vi "Facade.vi"(0 "Data In":T4, 2 "Display State In":T2, 3 "Container State":T3) -> (6 "Data Out":T4, 7 "Display State Out":T2, 8 "Action":T1)   [LabVIEW 2015, in "Moving Ripple Noise.xctl"]
uses:
  Moving Ripple Noise.xctl
  Data.vi
  Classes/Waveforms/Moving Ripple Noise/Moving Ripple Noise.lvclass
  <vilib>/_xctls/Container State.ctl
  State.vi
  <vilib>/_xctls/Action.ctl
  Classes/Waveforms/Moving Ripple Noise/Moving Ripple Noise.lvclass/Moving Ripple Noise.ctl
  Classes/Waveforms/Moving Ripple Noise/Read Fmin.vi
  Classes/Waveforms/Moving Ripple Noise/Read Fmax.vi
  Classes/Waveforms/Moving Ripple Noise/Read Comp_oct.vi
  Classes/Waveforms/Moving Ripple Noise/Read Density.vi
  Classes/Waveforms/Moving Ripple Noise/Read Velocity.vi
  Classes/Waveforms/Moving Ripple Noise/Read Depth.vi
  Classes/Waveforms/Moving Ripple Noise/Read Phase.vi
  Classes/Waveforms/Moving Ripple Noise/Write Fmin.vi
  Classes/Waveforms/Moving Ripple Noise/Write Fmax.vi
  Classes/Waveforms/Moving Ripple Noise/Write Comp_oct.vi
  Classes/Waveforms/Moving Ripple Noise/Write Density.vi
  Classes/Waveforms/Moving Ripple Noise/Write Velocity.vi
  Classes/Waveforms/Moving Ripple Noise/Write Depth.vi
  Classes/Waveforms/Moving Ripple Noise/Write Phase.vi
  <vilib>/_xctls/XControlSupport.lvlib
panel:
  in  "Plot":bool
  in  "Comp/oct":i32
  in  "Depth (0-1)":dbl
  in  "Velocity (Hz)":dbl
  in  "Density (cyc/oct)":dbl
  in  "Phase (cyc)":dbl
  in  "Fmin (Hz)":dbl
  in  "Fmax (Hz)":dbl
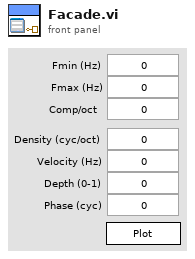
[diagram p1: front panel]
types:
  T1 = typedef "XControlSupport.lvlib/Action.ctl" = cluster{"Data Changed?":bool, "State Changed?":bool, "Action Name":string}
  T2 = typedef "Moving Ripple Noise.xctl/State.vi" = cluster{"Numeric":dbl}
  T3 = typedef "XControlSupport.lvlib/Container State.ctl" = cluster{"Indicator?":bool, "Run Mode?":bool, " Refnum":refnum<vi>}
  T4 = typedef "Moving Ripple Noise.xctl/Data.vi" = refnum<class "Moving Ripple Noise.lvclass">
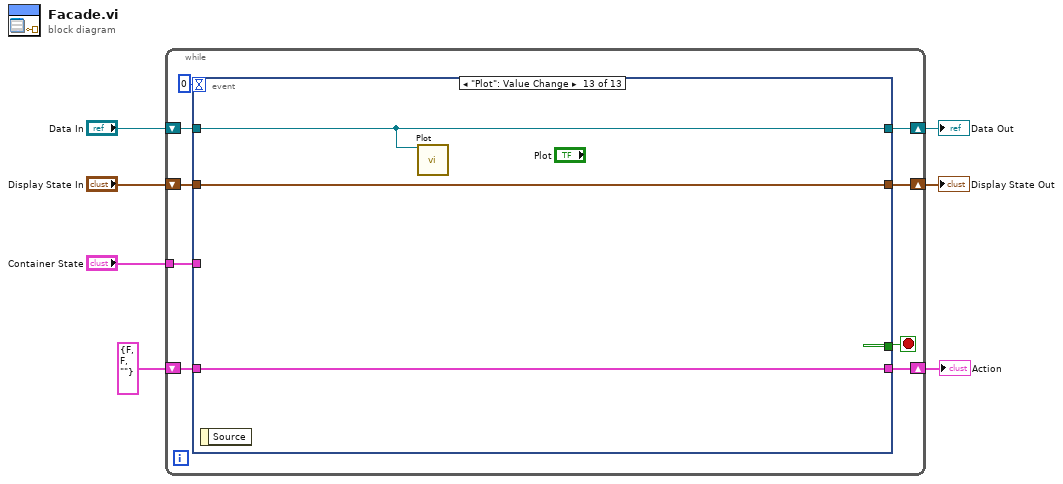
[diagram p0: block diagram]
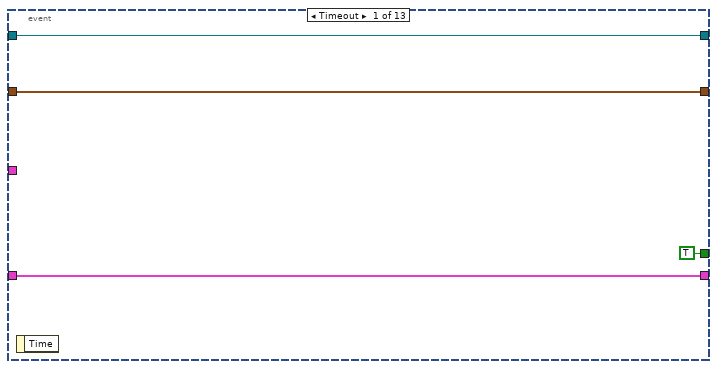
[diagram p2: hidden frame]
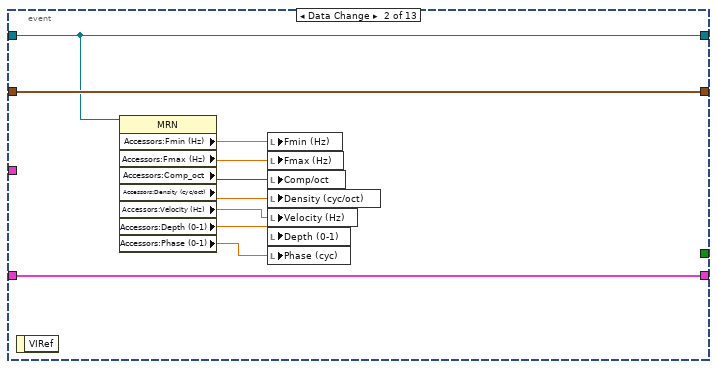
[diagram p3: hidden frame]
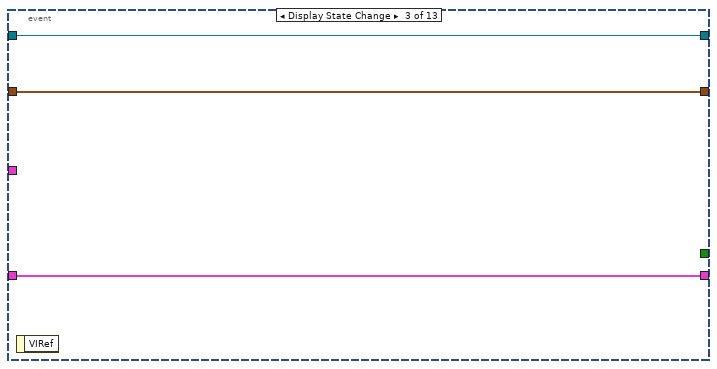
[diagram p4: hidden frame]
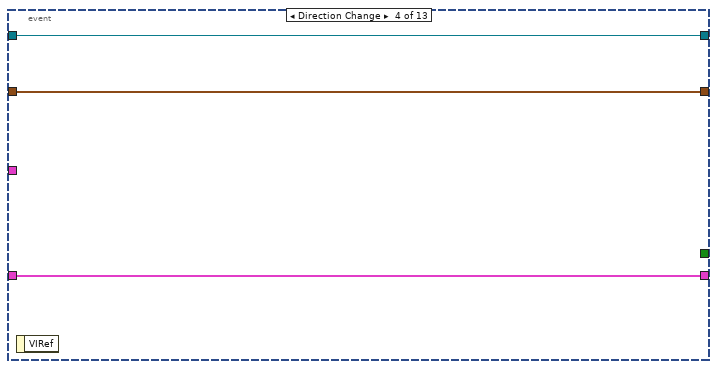
[diagram p5: hidden frame]
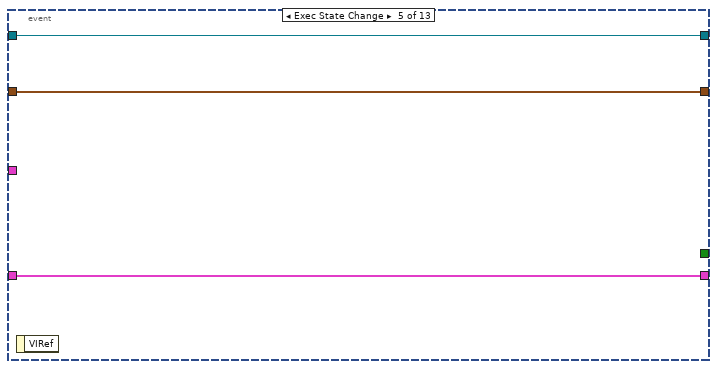
[diagram p6: hidden frame]
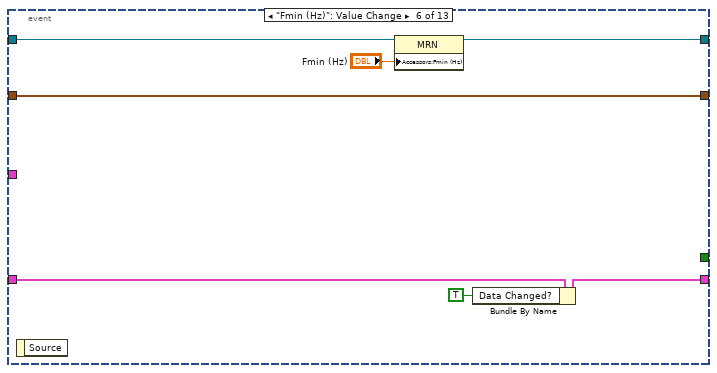
[diagram p7: hidden frame]
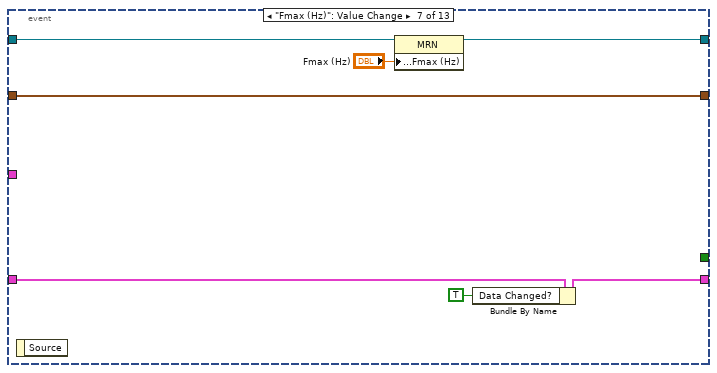
[diagram p8: hidden frame]
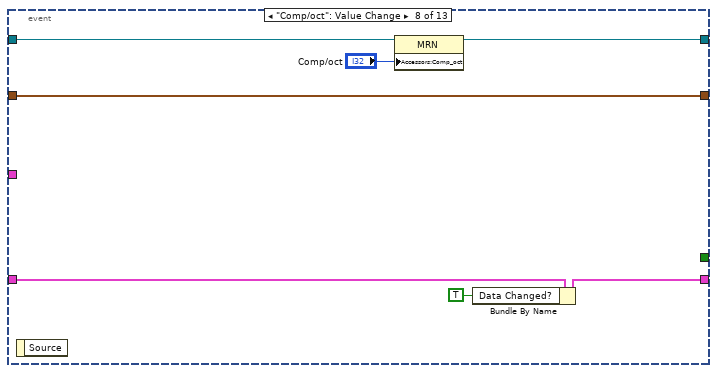
[diagram p9: hidden frame]
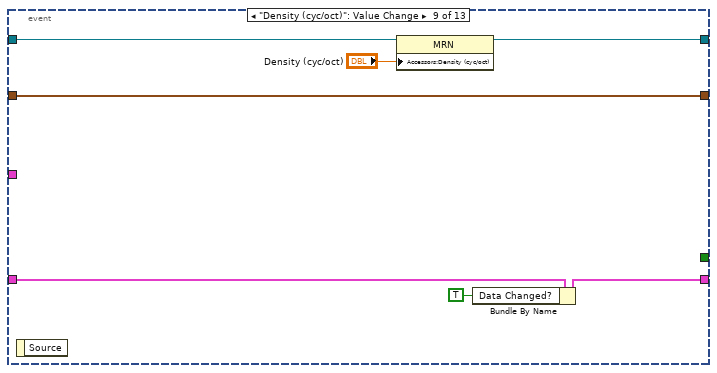
[diagram p10: hidden frame]
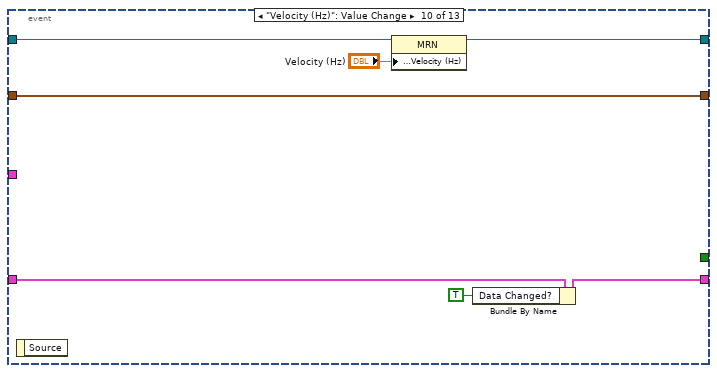
[diagram p11: hidden frame]
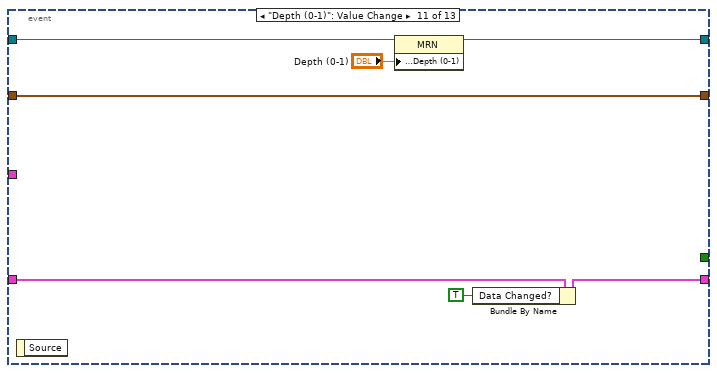
[diagram p12: hidden frame]
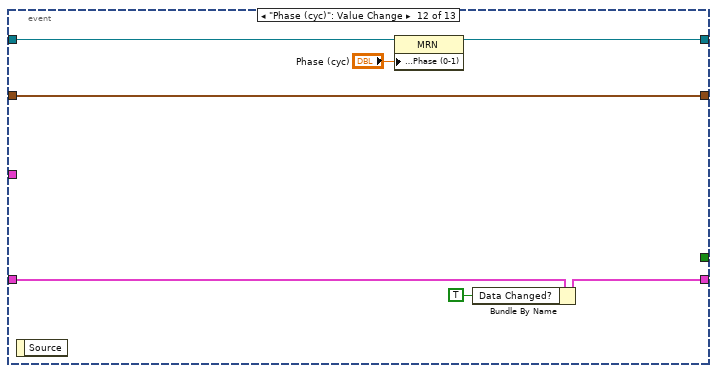
[diagram p13: hidden frame]
diagram:
  n1 = while {
    shift-right: [w15] -> w4
    shift-left: "Display State In" -> [w16]
    tunnel: "Container State" -> [w12]
    shift-right: [w10] -> w7
    shift-left: "Data In" -> [w11]
    shift-right: [w8] -> w2
    shift-left: T1 {"Data Changed?"=FALSE, "State Changed?"=FALSE, "Action Name"=""} ("Action") -> [w9]
    stop <- w14 stop-if-true
    n2 = event shown="[12] \"Plot\": Value Change" {
      selector: _ -> [_ _ _ _ _ _ _ _ _ _ _ _ _]
      dyn-events: _ -> [_ _ _ _ _ _ _ _ _ _ _ _ _]
      timeout: 0 -> [_ _ _ _ _ _ _ _ _ _ _ _ _]
      tunnel: w16 -> [w18 w30 w33 w36 w39 w46 w53 w60 w67 w74 w81 w88 w91]
      tunnel: [w18 w30 w33 w36 w39 w46 w53 w60 w67 w74 w81 w88 w91] -> w15
      tunnel: [TRUE _ _ _ _ _ _ _ _ _ _ _ _] -> w14
      tunnel: w12 -> [_ _ _ _ _ _ _ _ _ _ _ _ _]
      tunnel: w11 -> [w17 w28 w32 w35 w38 w45 w52 w59 w66 w73 w80 w87 w89]
      tunnel: [w17 w28 w32 w35 w38 w43 w50 w57 w64 w71 w78 w85 w89] -> w10
      tunnel: [w19 w29 w31 w34 w37 w42 w49 w56 w63 w70 w77 w84 w90] -> w8
      tunnel: w9 -> [w19 w29 w31 w34 w37 w44 w51 w58 w65 w72 w79 w86 w90]
      event Timeout {
        n3 = event-data() -> ()  [unwired: 1 in, 1 out]
      }
      event Data Change {
        n4 = event-data() -> ()  [unwired: 1 in, 1 out]
        n5 = property class="MRN"(reference=w28) -> ("Accessors:Fmin (Hz)"=w27:dbl, "Accessors:Fmax (Hz)"=w26:dbl, "Accessors:Comp_oct"=w25:i32, "Accessors:Density (cyc/oct)"=w24:dbl, "Accessors:Velocity (Hz)"=w23:dbl, "Accessors:Depth (0-1)"=w22:dbl, "Accessors:Phase (0-1)"=w21:dbl)  [unwired: 1 in, 2 out]
        n6 = local write "Fmin (Hz)"(w27) -> ()
        n7 = local write "Fmax (Hz)"(w26) -> ()
        n8 = local write "Comp/oct"(w25) -> ()
        n9 = local write "Density (cyc/oct)"(w24) -> ()
        n10 = local write "Velocity (Hz)"(w23) -> ()
        n11 = local write "Depth (0-1)"(w22) -> ()
        n12 = local write "Phase (cyc)"(w21) -> ()
      }
      event Display State Change {
        n13 = event-data() -> ()  [unwired: 1 in, 1 out]
      }
      event Direction Change {
        n14 = event-data() -> ()  [unwired: 1 in, 1 out]
      }
      event Exec State Change {
        n15 = event-data() -> ()  [unwired: 1 in, 1 out]
      }
      event "Fmin (Hz)": Value Change {
        n16 = event-data() -> ()  [unwired: 1 in, 1 out]
        n17 = property class="MRN"(reference=w45, "Accessors:Fmin (Hz)"="Fmin (Hz)") -> (reference out=w43:T4)  [unwired: 1 in, 1 out]
        n18 = Bundle By Name(cluster=w44, "Data Changed?"=TRUE) -> (w42:T1)
      }
      event "Fmax (Hz)": Value Change {
        n19 = event-data() -> ()  [unwired: 1 in, 1 out]
        n20 = property class="MRN"(reference=w52, "Accessors:Fmax (Hz)"="Fmax (Hz)") -> (reference out=w50:T4)  [unwired: 1 in, 1 out]
        n21 = Bundle By Name(cluster=w51, "Data Changed?"=TRUE) -> (w49:T1)
      }
      event "Comp/oct": Value Change {
        n22 = event-data() -> ()  [unwired: 1 in, 1 out]
        n23 = property class="MRN"(reference=w59, "Accessors:Comp_oct"="Comp/oct") -> (reference out=w57:T4)  [unwired: 1 in, 1 out]
        n24 = Bundle By Name(cluster=w58, "Data Changed?"=TRUE) -> (w56:T1)
      }
      event "Density (cyc/oct)": Value Change {
        n25 = event-data() -> ()  [unwired: 1 in, 1 out]
        n26 = property class="MRN"(reference=w66, "Accessors:Density (cyc/oct)"="Density (cyc/oct)") -> (reference out=w64:T4)  [unwired: 1 in, 1 out]
        n27 = Bundle By Name(cluster=w65, "Data Changed?"=TRUE) -> (w63:T1)
      }
      event "Velocity (Hz)": Value Change {
        n28 = event-data() -> ()  [unwired: 1 in, 1 out]
        n29 = property class="MRN"(reference=w73, "Accessors:Velocity (Hz)"="Velocity (Hz)") -> (reference out=w71:T4)  [unwired: 1 in, 1 out]
        n30 = Bundle By Name(cluster=w72, "Data Changed?"=TRUE) -> (w70:T1)
      }
      event "Depth (0-1)": Value Change {
        n31 = event-data() -> ()  [unwired: 1 in, 1 out]
        n32 = property class="MRN"(reference=w80, "Accessors:Depth (0-1)"="Depth (0-1)") -> (reference out=w78:T4)  [unwired: 1 in, 1 out]
        n33 = Bundle By Name(cluster=w79, "Data Changed?"=TRUE) -> (w77:T1)
      }
      event "Phase (cyc)": Value Change {
        n34 = event-data() -> ()  [unwired: 1 in, 1 out]
        n35 = property class="MRN"(reference=w87, "Accessors:Phase (0-1)"="Phase (cyc)") -> (reference out=w85:T4)  [unwired: 1 in, 1 out]
        n36 = Bundle By Name(cluster=w86, "Data Changed?"=TRUE) -> (w84:T1)
      }
      event "Plot": Value Change {
        n37 = event-data() -> ()  [unwired: 1 in, 1 out]
        n38 = call "Plot.vi"("MRN in"=w89) -> ()  [unwired: 13 in, 2 out]
      }
    }
  }
  "Display State Out" <- w4
  "Data Out" <- w7
  "Action" <- w2
